vi "LabViewTest.vi"() -> ()   [LabVIEW 2016]
panel:
  in  "Numeric":i32
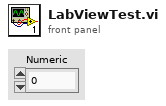
[diagram p1: front panel]
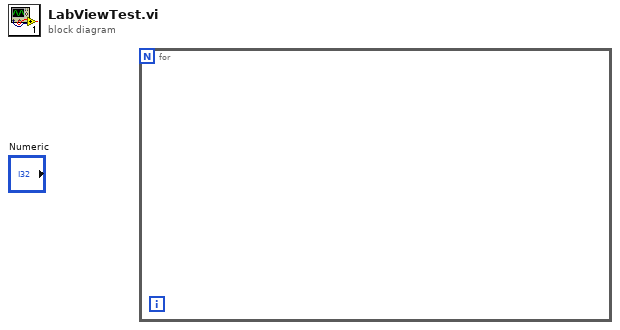
[diagram p0: block diagram]
diagram:
  n1 = for {
  }
